vi "161-Test QoS Repetition Bug.vi"() -> ()   [LabVIEW 2013]
uses:
  <vilib>/LabVIEW Open Source Project/MQTT Control Packets/Control Packets/CONNACK/Connect Return Code -- enum.ctl
  <vilib>/LabVIEW Open Source Project/MQTT Control Packets/Control Packets/ControlPacket/QualityOfService -- enum.ctl
  <vilib>/LabVIEW Open Source Project/MQTT Control Packets/Control Packets/CONNECT/ConnectFlags -- cluster.ctl
  source/Server class/Server.lvclass/Server.ctl
  <vilib>/LabVIEW Open Source Project/MQTT Client/Client class/Client.lvclass/Client.ctl
  <vilib>/LabVIEW Open Source Project/MQTT Control Packets/Control Packets/PUBLISH/PUBLISH.lvclass
  source/Server class/Server.lvclass
  <vilib>/LabVIEW Open Source Project/MQTT Connection/MQTT_Base/Base Class/MQTT_Base.lvclass
  <vilib>/LabVIEW Open Source Project/MQTT Client/Client class/Client.lvclass
  <vilib>/LabVIEW Open Source Project/MQTT TCP Connection/MQTT_TCP/Connection/TCPConnection.lvclass
  <vilib>/LabVIEW Open Source Project/MQTT LocalQueue Connection/MQTT_LocalQueue/Connection/LocalQueueConnection.lvclass
  <vilib>/LabVIEW Open Source Project/MQTT Websockets Connection/MQTT_Websockets/Connection/WebsocketsConnection.lvclass
  <vilib>/LabVIEW Open Source Project/MQTT Control Packets/Control Packets/CONNECT/CONNECT.lvclass
  <vilib>/LabVIEW Open Source Project/MQTT Control Packets/Control Packets/ControlPacket/ControlPacket.lvclass
  <vilib>/LabVIEW Open Source Project/MQTT Control Packets/Control Packets/CONNACK/CONNACK.lvclass
panel:
  out "FAILED":bool
  out "DUP":bool
  out "SubAck":bool
  in  "QoS Subscription":T1
  out "error server":errorcluster
  out "error client sink 2":errorcluster
  out "Random":dbl
  out "received 2":i32
  out "Client Status 2":T2=enum."Server Unavailable"
  out "error client source":errorcluster
  out "NbConnections":u32
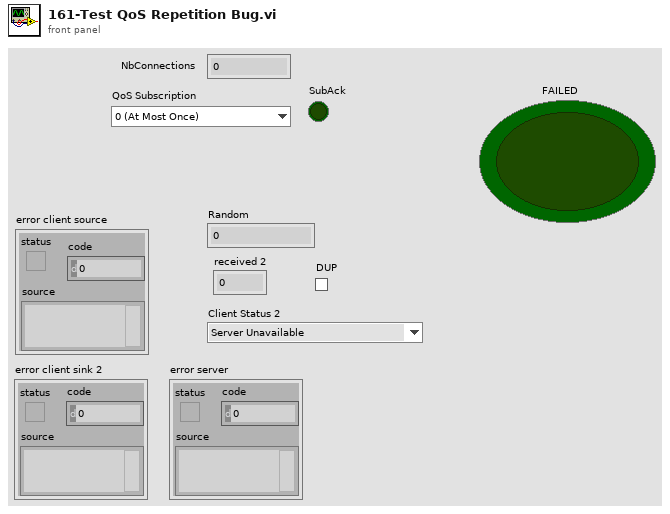
[diagram p1: front panel]
types:
  T1 = typedef "MQTT_Control_Packets.lvlib/ControlPacket.lvclass/QualityOfService -- enum.ctl" = enum16{"0 (At Most Once)", "1 (At Least Once)", "2 (Exactly Once)"}
  T2 = typedef "MQTT_Control_Packets.lvlib/CONNACK.lvclass/Connect Return Code -- enum.ctl" = enum16{"Connection accepted", "Unacceptable protocol version", "Identifier Rejected", "Server Unavailable", "Bad Username or Password", "Not Authorized"}
  T3 = typedef "MQTT_Control_Packets.lvlib/CONNECT.lvclass/ConnectFlags -- cluster.ctl" = cluster{"Reserved":bool, "Clean Session":bool, "Will Flag":bool, "Will QoS 1":bool, "Will QoS 2":bool, "Will Retain":bool, "Password Flag":bool, "User Name Flag":bool}
  T4 = typedef "MQTT Client.lvlib/Client.lvclass/Public Events -- cluster.ctl" = cluster{"Connection Status":refnum<user-event>, "Connected":refnum<user-event>, "Application Message":refnum<user-event>}
  T5 = typedef "MQTT Server.lvlib/Server.lvclass/Public Events -- cluster.ctl" = cluster{"NbConnections":refnum<user-event>}
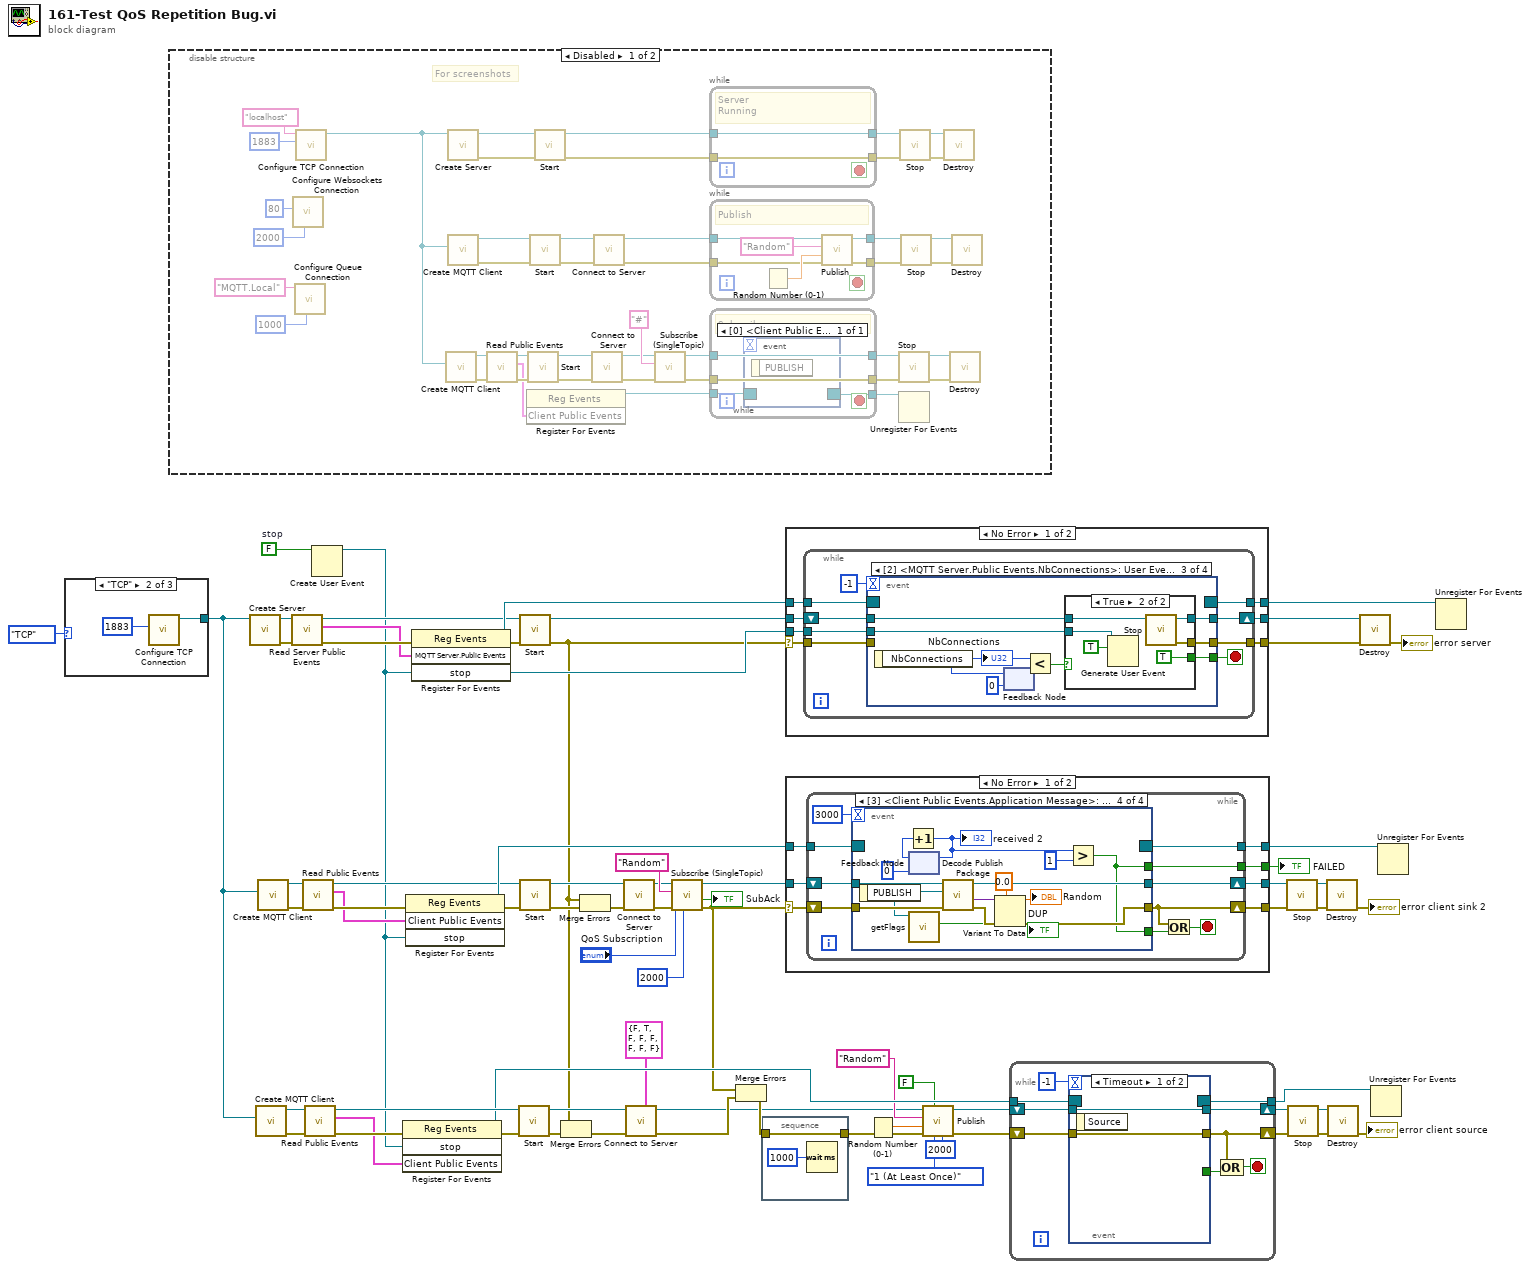
[diagram p0: block diagram]
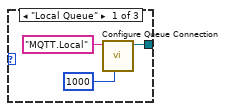
[diagram p2: hidden frame]
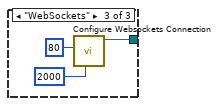
[diagram p3: hidden frame]
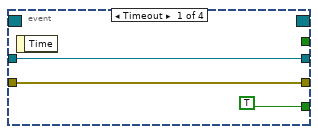
[diagram p5: hidden frame]
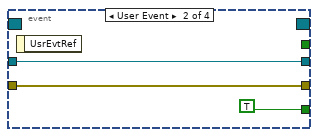
[diagram p6: hidden frame]
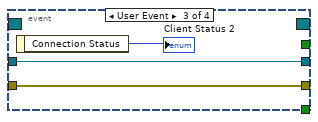
[diagram p7: hidden frame]
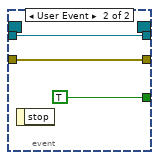
[diagram p9: hidden frame]
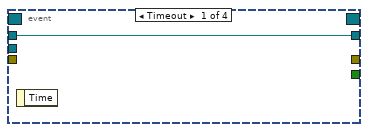
[diagram p10: hidden frame]
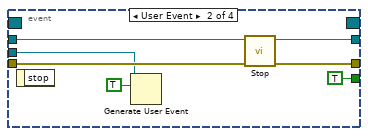
[diagram p11: hidden frame]
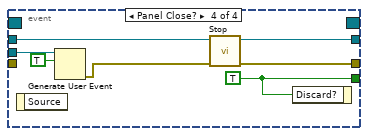
[diagram p13: hidden frame]
diagram:
  w48 = FALSE  # stop
  n1 = case shown="\"TCP\"" enum16{"TCP", "Local Queue", "WebSockets"}."TCP" ("Connection Type") {
    tunnel: [w71 w74 w78] -> w14
    frame "Local Queue" {
      n2 = call <vilib>:"Configure Queue Connection.vi"("timeout (500 ms)"=1000 ("timeout (100ms)"), "Queue Name"="MQTT.Local") -> ("LocalQueueConnection"=w71:refnum<class "LocalQueueConnection.lvclass">)  [unwired: 8 in, 1 out]
    }
    frame "TCP" {
      n3 = call <vilib>:"Configure TCP Connection.vi"("remote port (80)"=u16 1883) -> ("TCPConnection"=w74:refnum<class "TCPConnection.lvclass">)  [unwired: 9 in, 1 out]
    }
    frame "WebSockets" {
      n4 = call <vilib>:"Configure Websockets Connection.vi"("timeout (5000 ms)"=2000 ("timeout (100ms)"), "remote port (80)"=u16 80) -> ("WSConnection"=w78:refnum<class "WebsocketsConnection.lvclass">)  [unwired: 8 in, 1 out]
    }
  }
  n5 = disable-structure shown="Disabled" {
    frame Disabled {
      # "For screenshots"
      n6 = call <vilib>:"Configure Websockets Connection.vi"("timeout (5000 ms)"=2000 ("timeout (100ms)"), "remote port (80)"=u16 80) -> ()  [unwired: 8 in, 2 out]
      n7 = call <vilib>:"Configure Queue Connection.vi"("timeout (500 ms)"=1000 ("timeout (100ms)"), "Queue Name"="MQTT.Local") -> ()  [unwired: 8 in, 2 out]
      n8 = call <vilib>:"Configure TCP Connection.vi"("remote port (80)"=u16 1883, "address (localhost)"="localhost" ("Topic Filter")) -> ("TCPConnection"=w84:refnum<class "TCPConnection.lvclass">)  [unwired: 8 in, 1 out]
      n9 = call <vilib>:"Create MQTT Client.vi"("Connection Configuration"=w84) -> ("error out"=w90:errorcluster, "Client out"=w92:refnum<class "Client.lvclass">)  [unwired: 9 in]
      n10 = call "Create Server.vi"("Connection Configuration"=w84) -> ("error out"=w115:errorcluster, "Server"=w114:refnum<class "Server.lvclass">)  [unwired: 9 in]
      n11 = call <vilib>:"Create MQTT Client.vi"("Connection Configuration"=w84) -> ("error out"=w112:errorcluster, "Client out"=w113:refnum<class "Client.lvclass">)  [unwired: 9 in]
      n12 = call <vilib>:"Read Public Events.vi"("error in (no error)"=w90, "Client in"=w92) -> ("error out"=w89:errorcluster, "Client Public Events"=w88:T4, "Client out"=w91:refnum<class "Client.lvclass">)  [unwired: 7 in]
      n13 = register-events(w88) -> (reference out=w87:refnum<event-registration>)  [unwired: 2 in, 1 out]
      n14 = call <vilib>:"Start.vi"("error in (no error)"=w89, "MQTT_Base in"=w91) -> ("error out"=w107:errorcluster, "MQTT_Base out"=w108:refnum<class "Client.lvclass">)  [unwired: 7 in, 1 out]
      n15 = call <vilib>:"Start.vi"("error in (no error)"=w112, "MQTT_Base in"=w113) -> ("error out"=w119:errorcluster, "MQTT_Base out"=w118:refnum<class "Client.lvclass">)  [unwired: 7 in, 1 out]
      n16 = call <vilib>:"Start.vi"("error in (no error)"=w115, "MQTT_Base in"=w114) -> ("error out"=w99:errorcluster, "MQTT_Base out"=w101:refnum<class "Server.lvclass">)  [unwired: 7 in, 1 out]
      n17 = call <vilib>:"Connect to Server.vi"("error in (no error)"=w107, "Client in"=w108) -> ("error out"=w95:errorcluster, "Client out"=w96:refnum<class "Client.lvclass">)  [unwired: 6 in, 2 out]
      n18 = call <vilib>:"Connect to Server.vi"("error in (no error)"=w119, "Client in"=w118) -> ("error out"=w103:errorcluster, "Client out"=w106:refnum<class "Client.lvclass">)  [unwired: 6 in, 2 out]
      n19 = call <vilib>:"Subscribe (SingleTopic).vi"("error in (no error)"=w95, "Topic Filter"="#", "MQTT_Base in"=w96) -> ("error out"=w93:errorcluster, "MQTT_Base out"=w94:refnum<class "Client.lvclass">)  [unwired: 6 in, 1 out]
      n20 = while {
        tunnel: [w133] -> w102
        tunnel: w101 -> [w133]
        tunnel: w99 -> [w132]
        tunnel: [w132] -> w100
        stop <- _ stop-if-true
        # "Server\nRunning"
      }
      n21 = while {
        tunnel: w106 -> [w129]
        tunnel: [w128] -> w105
        tunnel: [w127] -> w104
        tunnel: w103 -> [w126]
        stop <- _ stop-if-true
        # "Publish"
        n22 = Random Number (0-1)() -> (number: 0 to 1=w131:dbl)
        n23 = call <vilib>:"Publish.vi"("error in (no error)"=w126, "Payload"=w131, "Topic Name (empty: Payload name)"="Random", "Client in"=w129) -> ("error out"=w127:errorcluster, "Client out"=w128:refnum<class "Client.lvclass">)  [unwired: 5 in, 1 out]
      }
      n24 = while {
        tunnel: [w125] -> w97
        tunnel: w94 -> [w125]
        tunnel: w93 -> [w124]
        tunnel: [w124] -> w98
        tunnel: w87 -> [w123]
        tunnel: [w122] -> w86
        stop <- _ stop-if-true
        # "Subscribe"
        n25 = event shown="[0] <Client Public Events.Application Message>: User Event" {
          selector: w123 -> [_]
          dyn-events: [_] -> w122
          timeout: _ -> [_]
          event User Event {
            n26 = event-data() -> ()  [unwired: 1 in, 1 out]
          }
        }
      }
      n27 = call <vilib>:"Stop.vi"("error in (no error)"=w98, "MQTT_Base in"=w97) -> ("error out"=w110:errorcluster, "MQTT_Base out"=w111:refnum<class "Client.lvclass">)  [unwired: 7 in, 1 out]
      n28 = Unregister For Events(event registration refnum=w86) -> ()  [unwired: 1 in, 1 out]
      n29 = call <vilib>:"Stop.vi"("error in (no error)"=w100, "MQTT_Base in"=w102) -> ("error out"=w121:errorcluster, "MQTT_Base out"=w120:refnum<class "Server.lvclass">)  [unwired: 7 in, 1 out]
      n30 = call <vilib>:"Stop.vi"("error in (no error)"=w104, "MQTT_Base in"=w105) -> ("error out"=w117:errorcluster, "MQTT_Base out"=w116:refnum<class "Client.lvclass">)  [unwired: 7 in, 1 out]
      n31 = call <vilib>:"Destroy.vi"("error in (no error)"=w121, "MQTT_Base in"=w120) -> ()  [unwired: 8 in, 2 out]
      n32 = call <vilib>:"Destroy.vi"("error in (no error)"=w110, "MQTT_Base in"=w111) -> ()  [unwired: 8 in, 2 out]
      n33 = call <vilib>:"Destroy.vi"("error in (no error)"=w117, "MQTT_Base in"=w116) -> ()  [unwired: 8 in, 2 out]
    }
    frame Enabled {
    }
  }
  n34 = call "Create Server.vi"("Connection Configuration"=w14) -> ("error out"=w68:errorcluster, "Server"=w69:refnum<class "Server.lvclass">)  [unwired: 9 in]
  n35 = call <vilib>:"Create MQTT Client.vi"("Connection Configuration"=w14) -> ("error out"=w57:errorcluster, "Client out"=w56:refnum<class "Client.lvclass">)  [unwired: 9 in]
  n36 = call <vilib>:"Create MQTT Client.vi"("Connection Configuration"=w14) -> ("error out"=w25:errorcluster, "Client out"=w24:refnum<class "Client.lvclass">)  [unwired: 9 in]
  n37 = call "Read Server Public Events.vi"("error in (no error)"=w68, "Server in"=w69) -> ("error out"=w67:errorcluster, "MQTT Server.Public Events"=w66:T5, "Server out"=w63:refnum<class "Server.lvclass">)  [unwired: 7 in]
  n38 = call <vilib>:"Read Public Events.vi"("error in (no error)"=w25, "Client in"=w24) -> ("error out"=w35:errorcluster, "Client Public Events"=w34:T4, "Client out"=w26:refnum<class "Client.lvclass">)  [unwired: 7 in]
  n39 = call <vilib>:"Read Public Events.vi"("error in (no error)"=w57, "Client in"=w56) -> ("error out"=w47:errorcluster, "Client Public Events"=w43:T4, "Client out"=w55:refnum<class "Client.lvclass">)  [unwired: 7 in]
  n40 = Create User Event(user event datatype=w48) -> (user event=w21:refnum<user-event>)  [unwired: 1 in, 1 out]
  n41 = register-events(error in=w47, w21, w43) -> (reference out=w45:refnum<event-registration>, error out=w46:errorcluster)  [unwired: 1 in]
  n42 = register-events(error in=w35, w34, w21) -> (reference out=w37:refnum<event-registration>, error out=w36:errorcluster)  [unwired: 1 in]
  n43 = register-events(error in=w67, w66, w21) -> (reference out=w65:refnum<event-registration>, error out=w61:errorcluster)  [unwired: 1 in]
  n44 = call <vilib>:"Start.vi"("error in (no error)"=w46, "MQTT_Base in"=w55) -> ("error out"=w53:errorcluster, "MQTT_Base out"=w54:refnum<class "Client.lvclass">)  [unwired: 7 in, 1 out]
  n45 = call <vilib>:"Start.vi"("error in (no error)"=w61, "MQTT_Base in"=w63) -> ("error out"=w20:errorcluster, "MQTT_Base out"=w62:refnum<class "Server.lvclass">)  [unwired: 7 in, 1 out]
  n46 = call <vilib>:"Start.vi"("error in (no error)"=w36, "MQTT_Base in"=w26) -> ("error out"=w28:errorcluster, "MQTT_Base out"=w27:refnum<class "Client.lvclass">)  [unwired: 7 in, 1 out]
  n47 = Merge Errors(w20, w53) -> (w58:errorcluster)
  n48 = Merge Errors(w20, w28) -> (w23:errorcluster)
  n49 = call <vilib>:"Connect to Server.vi"("error in (no error)"=w23, "Client in"=w27) -> ("error out"=w32:errorcluster, "Client out"=w31:refnum<class "Client.lvclass">)  [unwired: 6 in, 2 out]
  n50 = call <vilib>:"Connect to Server.vi"("Connect Flags"=T3 {"Reserved"=FALSE, "Clean Session"=TRUE, "Will Flag"=FALSE, "Will QoS 1"=FALSE, "Will QoS 2"=FALSE, "Will Retain"=FALSE, "Password Flag"=FALSE, "User Name Flag"=FALSE}, "error in (no error)"=w58, "Client in"=w54) -> ("error out"=w42:errorcluster, "Client out"=w4:refnum<class "Client.lvclass">)  [unwired: 5 in, 2 out]
  n51 = call <vilib>:"Subscribe (SingleTopic).vi"("timeout (100ms)"=2000, "error in (no error)"=w32, "QoS"="QoS Subscription", "Topic Filter"="Random", "MQTT_Base in"=w31) -> ("error out"=w19:errorcluster, "Ack"=→"SubAck":bool, "MQTT_Base out"=w39:refnum<class "Client.lvclass">)  [unwired: 4 in]
  n52 = Merge Errors(w19, w42) -> (w49:errorcluster)
  n53 = stacked-sequence {
    tunnel: [w134] -> w5
    tunnel: w49 -> [w134]
    frame #0 {
      n54 = Wait (ms)(milliseconds to wait=u32 1000) -> ()  [unwired: 1 out]
    }
  }
  n55 = case shown="No Error" w20 {
    selector: w20 -> [w136 w183]
    tunnel: w62 -> [w142 w185]
    tunnel: [w141 w185] -> w70
    tunnel: w65 -> [w140 w184]
    tunnel: [w139 w184] -> w64
    tunnel: [w138 w183] -> w60
    tunnel: w21 -> [w137 _]
    frame No Error {
      n56 = while {
        shift-right: [w148] -> w141
        shift-left: w142 -> [w150]
        tunnel: w140 -> [w147]
        tunnel: [w146] -> w139
        tunnel: [w145] -> w138
        tunnel: w137 -> [w144]
        tunnel: w136 -> [w143]
        stop <- w149 stop-if-true
        n57 = event shown="[2] <MQTT Server.Public Events.NbConnections>: User Event" {
          selector: w147 -> [_ _ _ _]
          dyn-events: [_ _ _ _] -> w146
          timeout: -1 -> [_ _ _ _]
          tunnel: w150 -> [w152 w159 w165 w182]
          tunnel: [_ TRUE ("Discard?") w161 w181] -> w149
          tunnel: [w152 w158 w164 w180] -> w148
          tunnel: [_ w157 w163 w179] -> w145
          tunnel: w144 -> [_ w153 w160 w178]
          tunnel: w143 -> [_ w155 _ _]
          event Timeout {
            n58 = event-data() -> ()  [unwired: 1 in, 1 out]
          }
          event User Event {
            n59 = event-data() -> ()  [unwired: 1 in, 1 out]
            n60 = Generate User Event(user event=w153, event data cluster=TRUE ("event data")) -> ()  [unwired: 2 in, 2 out]
            n61 = call <vilib>:"Stop.vi"("error in (no error)"=w155, "MQTT_Base in"=w159) -> ("error out"=w157:errorcluster, "MQTT_Base out"=w158:refnum<class "Server.lvclass">)  [unwired: 7 in, 1 out]
          }
          event User Event {
            n62 = event-data() -> ("NbConnections"=w167:u32)  [unwired: 1 in]
            "NbConnections" <- w167
            n63 = feedback #1(u32 0 ("NbConnections")) -> (w166:u32)
            n64 = feedback-in #1(w167) -> ()
            n65 = Less?(x=w167, y=w166) -> (x < y?=w162:bool)
            n66 = case shown="True" w162 {
              tunnel: w165 -> [w169 w175]
              tunnel: [w169 w174] -> w164
              tunnel: [_ w173] -> w163
              tunnel: [_ TRUE] -> w161
              tunnel: w160 -> [_ w170]
              frame False {
              }
              frame True {
                n67 = Generate User Event(user event=w170, event data cluster=TRUE ("event data")) -> ()  [unwired: 2 in, 2 out]
                n68 = call <vilib>:"Stop.vi"("MQTT_Base in"=w175) -> ("error out"=w173:errorcluster, "MQTT_Base out"=w174:refnum<class "Server.lvclass">)  [unwired: 8 in, 1 out]
              }
            }
          }
          event Panel Close? {
            w181 = TRUE ("Discard?")
            n69 = event-data() -> ()  [unwired: 1 in, 1 out]
            n70 = Generate User Event(user event=w178, event data cluster=TRUE ("event data")) -> (error out=w176:errorcluster)  [unwired: 2 in, 1 out]
            n71 = call <vilib>:"Stop.vi"("error in (no error)"=w176, "MQTT_Base in"=w182) -> ("error out"=w179:errorcluster, "MQTT_Base out"=w180:refnum<class "Server.lvclass">)  [unwired: 7 in, 1 out]
            n72 = event-data("Discard?"=w181) -> ()  [unwired: 1 in, 1 out]
          }
        }
      }
    }
    frame Error {
    }
  }
  n73 = case shown="No Error" w19 {
    selector: w19 -> [w187 w227]
    tunnel: w37 -> [w192 w229]
    tunnel: [w191 w229] -> w38
    tunnel: w39 -> [w190 w228]
    tunnel: [w189 w228] -> w40
    tunnel: [w188 w227] -> w41
    tunnel: [w186 _] -> w1
    frame No Error {
      n74 = while {
        tunnel: w192 -> [w202]
        tunnel: [w201] -> w191
        shift-right: [w199] -> w189
        shift-left: w190 -> [w200]
        shift-right: [w196] -> w188
        shift-left: w187 -> [w198]
        tunnel: [w193] -> w186
        stop <- w197 stop-if-true
        n75 = event shown="[3] <Client Public Events.Application Message>: User Event" {
          selector: w202 -> [_ _ _ _]
          dyn-events: [_ _ _ _] -> w201
          timeout: 3000 -> [_ _ _ _]
          tunnel: w200 -> [w204 w207 w210 w226]
          tunnel: [w204 w207 w210 w222] -> w199
          tunnel: [w203 w206 w209 w217] -> w196
          tunnel: w198 -> [w203 w206 w209 w221]
          tunnel: [TRUE TRUE _ w212] -> w195
          tunnel: [_ _ _ w212] -> w193
          event Timeout {
            n76 = event-data() -> ()  [unwired: 1 in, 1 out]
          }
          event User Event {
            n77 = event-data() -> ()  [unwired: 1 in, 1 out]
          }
          event User Event {
            n78 = event-data() -> ("Connection Status"=→"Client Status 2":T2)  [unwired: 1 in]
          }
          event User Event {
            n79 = event-data() -> ("PUBLISH"=w216:refnum<class "PUBLISH.lvclass">)  [unwired: 1 in]
            n80 = feedback #2(0 ("received")) -> (w219:i32)
            n81 = Increment(x=w219) -> (x+1=w214:i32)
            "received 2" <- w214
            n82 = feedback-in #2(w214) -> ()
            n83 = call-dynamic "getFlags.vi"("PUBLISH in"=w216) -> ("DUP"=→"DUP":bool)  [unwired: 7 in, 3 out]
            n84 = call <vilib>:"Decode Publish Package.vi"("error in (no error)"=w221, "PUBLISH"=w216, "MQTT_Base in"=w226) -> ("error out"=w218:errorcluster, "Payload"=w225:variant, "MQTT_Base out"=w222:refnum<class "Client.lvclass">)  [unwired: 5 in, 1 out]
            n85 = Variant To Data(error in=w218, type=0.0, Variant=w225) -> (data=→"Random":dbl, error out=w217:errorcluster)
            n86 = Greater?(x=w214, y=1) -> (0:w212:bool)
          }
        }
        n87 = Or(x=w196, y=w195) -> (x .or. y?=w197:bool)
      }
    }
    frame Error {
    }
  }
  "FAILED" <- w1
  n88 = Random Number (0-1)() -> (number: 0 to 1=w9:dbl)
  n89 = call <vilib>:"Publish.vi"("timeout (1000ms)"=2000, "QoS"=QualityOfService_--_enum."1 (At Least Once)" ("QoS Publication"), "DUP (Re-delivery attempt)"=FALSE, "error in (no error)"=w5, "Payload"=w9, "Topic Name (empty: Payload name)"="Random", "Client in"=w4) -> ("error out"=w6:errorcluster, "Client out"=w3:refnum<class "Client.lvclass">)  [unwired: 2 in, 1 out]
  n90 = while {
    shift-right: [w237] -> w52
    shift-left: w3 -> [w238]
    shift-right: [w230] -> w44
    shift-left: w6 -> [w236]
    tunnel: w45 -> [w234]
    tunnel: [w232] -> w18
    stop <- w235 stop-if-true
    n91 = event shown="[0] Timeout" {
      selector: w234 -> [_ _]
      dyn-events: [_ _] -> w232
      timeout: -1 -> [_ _]
      tunnel: w238 -> [w240 w241]
      tunnel: [w240 w241] -> w237
      tunnel: w236 -> [w239 w242]
      tunnel: [w239 w242] -> w230
      tunnel: [_ TRUE] -> w233
      event Timeout {
        n92 = event-data() -> ()  [unwired: 1 in, 1 out]
      }
      event User Event {
        n93 = event-data() -> ()  [unwired: 1 in, 1 out]
      }
    }
    n94 = Compound Arithmetic op=OR(w230, w233) -> (w235:bool)
  }
  n95 = call <vilib>:"Stop.vi"("error in (no error)"=w41, "MQTT_Base in"=w40) -> ("error out"=w29:errorcluster, "MQTT_Base out"=w30:refnum<class "Client.lvclass">)  [unwired: 7 in, 1 out]
  n96 = call <vilib>:"Stop.vi"("error in (no error)"=w44, "MQTT_Base in"=w52) -> ("error out"=w50:errorcluster, "MQTT_Base out"=w51:refnum<class "Client.lvclass">)  [unwired: 7 in, 1 out]
  n97 = call <vilib>:"Destroy.vi"("error in (no error)"=w29, "MQTT_Base in"=w30) -> ("error out"=→"error client sink 2":errorcluster)  [unwired: 8 in, 1 out]
  n98 = call <vilib>:"Destroy.vi"("error in (no error)"=w50, "MQTT_Base in"=w51) -> ("error out"=→"error client source":errorcluster)  [unwired: 8 in, 1 out]
  n99 = call <vilib>:"Destroy.vi"("error in (no error)"=w60, "MQTT_Base in"=w70) -> ("error out"=→"error server":errorcluster)  [unwired: 8 in, 1 out]
  n100 = Unregister For Events(event registration refnum=w18) -> ()  [unwired: 1 in, 1 out]
  n101 = Unregister For Events(event registration refnum=w38) -> ()  [unwired: 1 in, 1 out]
  n102 = Unregister For Events(event registration refnum=w64) -> ()  [unwired: 1 in, 1 out]
